vi "1_02.vi"() -> ()   [LabVIEW 2013]
panel:
  out "Indicador LED":bool
  in  "Boolean":bool
  out "Indicador de Cadena":string
  in  "Control de Cadena":string
  out "Indicador Numerico Flotante":dbl
  out "Indicador Numerico Entero":i32
  in  "Control Numerico Flotante":dbl
  in  "Control Numerico Enero":i32
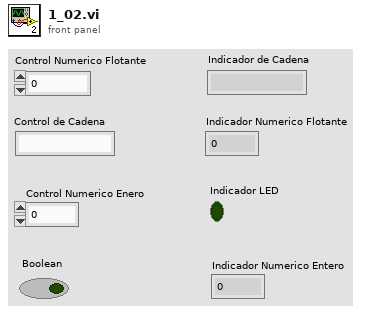
[diagram p1: front panel]
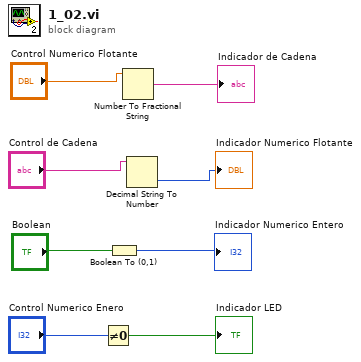
[diagram p0: block diagram]
diagram:
  n1 = Not Equal To 0?(x="Control Numerico Enero") -> (x != 0?=→"Indicador LED":bool)
  n2 = Boolean To (0,1)(Boolean="Boolean") -> (0, 1=→"Indicador Numerico Entero":i16)
  n3 = Number To Fractional String(number="Control Numerico Flotante") -> (F-format string=→"Indicador de Cadena":string)  [unwired: 3 in]
  n4 = Decimal String To Number(string="Control de Cadena") -> (number=→"Indicador Numerico Flotante":i32)  [unwired: 2 in, 1 out]
